vi "Vision Research Phantom Series PhCon PhBlackReferenceCI.vi"(0 "CN in":u32=1, 5 "Error In (no error)":errorcluster, 9 "CallID":u32) -> (14 "CN out":u32=1, 19 "Error Out":errorcluster)   [LabVIEW 2013, in "VRI.lvlib"]
doc: "PhCon.dll\n\nPhBlackReferenceCI\nHRESULT PhBlackReferenceCI(UINT CN, UINT CallID)\n\nParameters Description\nCN (in) Camera number.\nCallID (in) The call identifier (a number 1 to 15).\n Used as a progress indicator parameter \n for calling PhLVProgress().\nReturn HRESULT (0 = Ok)\nComments You have to ask the operator to cover the lenses before\n calling this function. A number of images will be\n acquired in the darkness, at the current acquisition\n parameters and the pixels offset will be computed and\n stored in the internal tables. This calibration is good\n only at the current parameters. To apply the calibration\n to the Video Out too, call the function PhWriteStgFlash."
uses:
  VRI.lvlib
  Phantom DLLs/PhCon.Dll
panel:
  # "For instructions on the use of this VI, press Ctrl+H to display the help window and move the mouse over the icon, controls, and indicators"
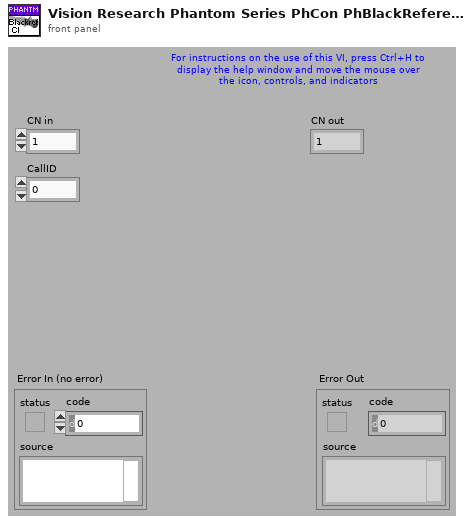
[diagram p1: front panel]
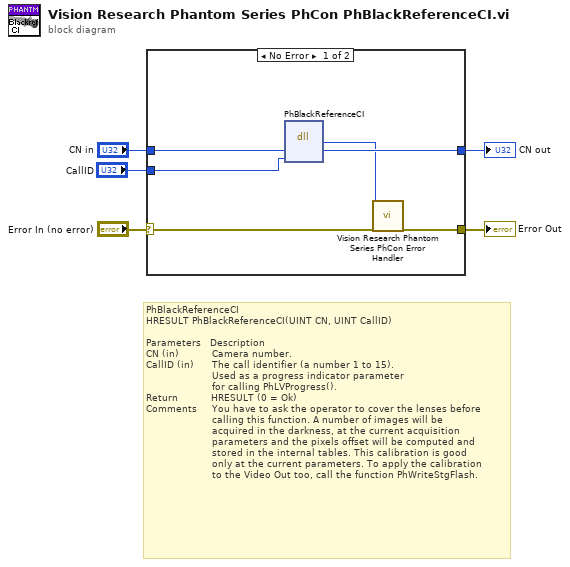
[diagram p0: block diagram]
diagram:
  # "PhBlackReferenceCI\nHRESULT PhBlackReferenceCI(UINT CN, UINT CallID)\n\nParameters   Description\nCN (in)           Camera number.\nCallID (in)      The call identifier (a number 1 to 15).\n                      Used as a progress indicator parameter \n                      for calling PhLVProgress().\nReturn           HRESULT (0 = Ok)\nComments     You have to ask the operator to cover the lenses before\n                      calling this function. A number of images will be\n                      acquired in the darkness, at the current acquisition\n                      parameters and the pixels offset will be computed and\n                      stored in the internal tables. This calibration is good\n                      only at the current parameters. To apply the calibration\n                      to the Video Out too, call the function PhWriteStgFlash."
  n1 = case shown="No Error" "Error In (no error)" {
    selector: "Error In (no error)" -> [w11 w13]
    tunnel: [w10 w13] -> w4
    tunnel: "CN in" -> [w9 w12]
    tunnel: [w8 w12] -> w2
    tunnel: "CallID" -> [w7 _]
    frame No Error {
      n2 = dll-call lib="C:/Projects/SDK/64-bit/Vision Research Phantom Series Labview Driver/Phantom DLLs/PhCon.dll" fn="PhBlackReferenceCI"("CN"=w9, "CallID"=w7) -> ("HRESULT"=w6:i32, "CN"=w8:u32)  [unwired: 4 in, 2 out]
      n3 = call "Vision Research Phantom Series PhCon Error Handler.vi"("ErrNo"=w6, "Error In (no error)"=w11) -> ("Error Out"=w10:errorcluster)  [unwired: 17 out]
    }
    frame Error {
    }
  }
  "Error Out" <- w4
  "CN out" <- w2
